vi "ReadData_6_modules.vi"(8 "error in":errorcluster, 11 "Module Config Selector":i16) -> (0 "error out":errorcluster, 1 "Number Of Pulses":u32, 2 "OversampleClk Ticks":u32, 3 "Data Array":sgl[](array[numeric]) format="%.2f")   [LabVIEW 2017, in "VDMS_VibAPI.lvlib"]
uses:
  <vilib>/addons/InsightCM/Devices/Shared/Cms/Fpga/AcquisitionFpgaTach/source/subVIs/VibAPI/VDMS_VibAPI.lvlib
  <vilib>/rvi/eio/common/nirviEmuTemplateMethod_errors.vi
  <vilib>/rvi/Memory/Memory_Emulation/nirvimemoryFastEmulation.vi
  <vilib>/rvi/Memory/Memory_Emulation/nirvimemoryEmulation.vi
  <vilib>/rvi/Emulation/niFpgaEmulationIsFPGAContextNoSignature.vi
  <vilib>/rvi/DataTransferAndStorage/Container/Common/niFpgaContainerGetUniqueNameForEmu.vi
  <vilib>/rvi/Emulation/niFpgaProcessEmulError.vi
  <vilib>/rvi/Emulation/niFpgaSctlEmulationGetInTimedLoop.vi
  <vilib>/rvi/errors/nirviReportUnexpectedCaseInternalError (U32).vi
  <vilib>/eio/EIONode/EIONode.xnode
  <vilib>/rvi/DataTransferAndStorage/Container/XNode/niFpgaContainer.xnode
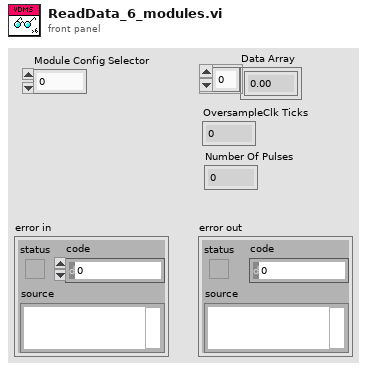
[diagram p1: front panel]
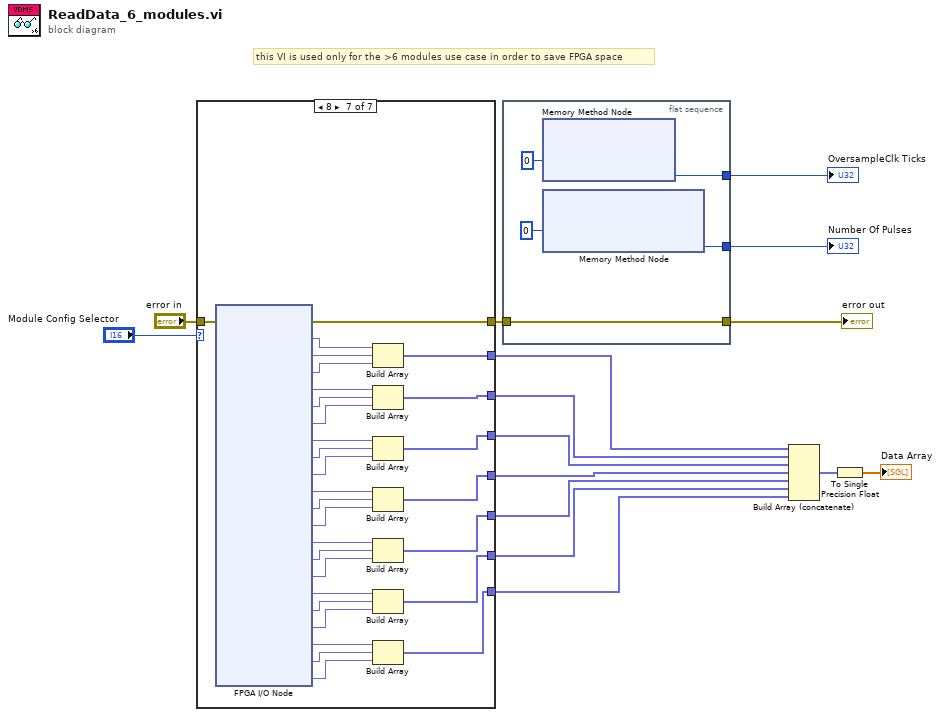
[diagram p0: block diagram]
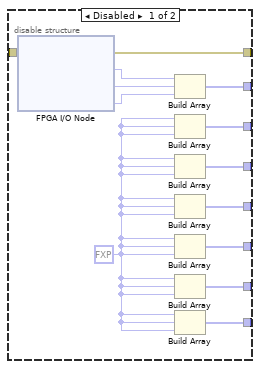
[diagram p3: hidden frame]
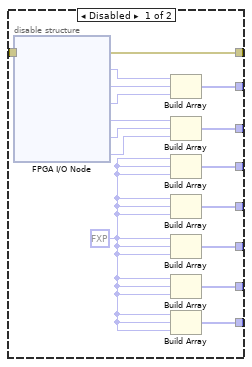
[diagram p5: hidden frame]
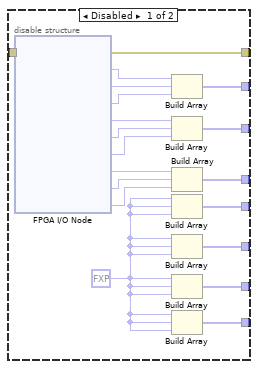
[diagram p7: hidden frame]
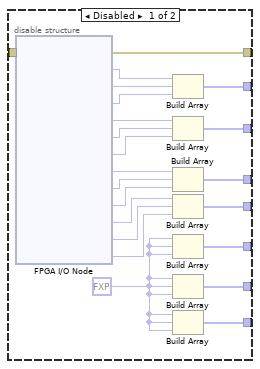
[diagram p9: hidden frame]
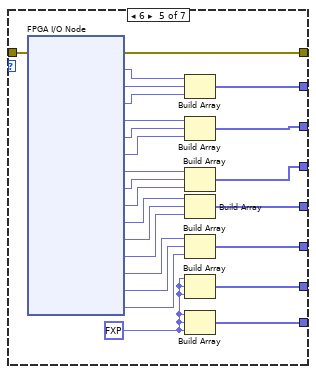
[diagram p10: hidden frame]
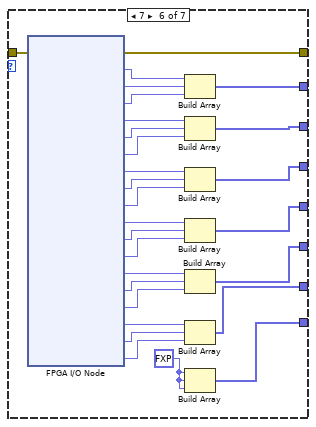
[diagram p11: hidden frame]
diagram:
  # "this VI is used only for the >6 modules use case in order to save FPGA space"
  n1 = case shown="8" "Module Config Selector" {
    tunnel: "error in" -> [w24 w47 w73 w102 w150 w178 w208]
    tunnel: [w23 w46 w72 w101 w149 w177 w207] -> w6
    tunnel: [w22 w45 w71 w100 w148 w176 w206] -> w14
    tunnel: [w21 w44 w70 w99 w147 w175 w205] -> w13
    tunnel: [w20 w43 w69 w98 w146 w174 w204] -> w12
    tunnel: [w19 w42 w68 w97 w145 w173 w203] -> w11
    tunnel: [w18 w41 w67 w96 w144 w172 w202] -> w10
    tunnel: [w17 w40 w66 w95 w143 w171 w201] -> w8
    tunnel: [w16 w39 w65 w94 w142 w170 w200] -> w7
    frame 2, Default {
      n2 = disable-structure shown="Enabled" {
        disable-tunnel: w24 -> [w37 w38]
        disable-tunnel: [w36 w38] -> w23
        disable-tunnel: [w35 _] -> w22
        disable-tunnel: [w34 _] -> w21
        disable-tunnel: [w33 _] -> w20
        disable-tunnel: [w32 _] -> w19
        disable-tunnel: [w31 _] -> w18
        disable-tunnel: [w27 _] -> w17
        disable-tunnel: [w25 _] -> w16
        frame Disabled {
          w26 = fxp<+/-,24,7> 0.0 ("Mod1/AI2")
          n3 = xnode "FPGA I/O Node"("error in"=w37) -> ("error out"=w36:errorcluster, "Mod2/AI0"=w30:fxp<+/-,24,7>, "Mod2/AI1"=w29:fxp<+/-,24,7>, "Mod2/AI2"=w28:fxp<+/-,24,7>)  [unwired: 3 in, 3 out]
          n4 = Build Array(w30, w29, w28) -> (w35:fxp<+/-,24,7>[])
          n5 = Build Array(w26, w26, w26) -> (w34:fxp<+/-,24,7>[])
          n6 = Build Array(w26, w26, w26) -> (w33:fxp<+/-,24,7>[])
          n7 = Build Array(w26, w26, w26) -> (w32:fxp<+/-,24,7>[])
          n8 = Build Array(w26, w26, w26) -> (w31:fxp<+/-,24,7>[])
          n9 = Build Array(w26, w26, w26) -> (w27:fxp<+/-,24,7>[])
          n10 = Build Array(w26, w26, w26) -> (w25:fxp<+/-,24,7>[])
        }
        frame Enabled {
        }
      }
    }
    frame 3 {
      n11 = disable-structure shown="Enabled" {
        disable-tunnel: w47 -> [w63 w64]
        disable-tunnel: [w62 w64] -> w46
        disable-tunnel: [w61 _] -> w45
        disable-tunnel: [w60 _] -> w44
        disable-tunnel: [w59 _] -> w43
        disable-tunnel: [w58 _] -> w42
        disable-tunnel: [w57 _] -> w41
        disable-tunnel: [w50 _] -> w40
        disable-tunnel: [w48 _] -> w39
        frame Disabled {
          w49 = fxp<+/-,24,7> 0.0 ("Mod1/AI2")
          n12 = xnode "FPGA I/O Node"("error in"=w63) -> ("error out"=w62:errorcluster, "Mod2/AI0"=w56:fxp<+/-,24,7>, "Mod2/AI1"=w55:fxp<+/-,24,7>, "Mod2/AI2"=w54:fxp<+/-,24,7>, "Mod3/AI0"=w53:fxp<+/-,24,7>, "Mod3/AI1"=w52:fxp<+/-,24,7>, "Mod3/AI2"=w51:fxp<+/-,24,7>)  [unwired: 6 in, 6 out]
          n13 = Build Array(w56, w55, w54) -> (w61:fxp<+/-,24,7>[])
          n14 = Build Array(w53, w52, w51) -> (w60:fxp<+/-,24,7>[])
          n15 = Build Array(w49, w49, w49) -> (w59:fxp<+/-,24,7>[])
          n16 = Build Array(w49, w49, w49) -> (w58:fxp<+/-,24,7>[])
          n17 = Build Array(w49, w49, w49) -> (w57:fxp<+/-,24,7>[])
          n18 = Build Array(w49, w49, w49) -> (w50:fxp<+/-,24,7>[])
          n19 = Build Array(w49, w49, w49) -> (w48:fxp<+/-,24,7>[])
        }
        frame Enabled {
        }
      }
    }
    frame 4 {
      n20 = disable-structure shown="Enabled" {
        disable-tunnel: w73 -> [w92 w93]
        disable-tunnel: [w91 w93] -> w72
        disable-tunnel: [w90 _] -> w71
        disable-tunnel: [w89 _] -> w70
        disable-tunnel: [w88 _] -> w69
        disable-tunnel: [w87 _] -> w68
        disable-tunnel: [w86 _] -> w67
        disable-tunnel: [w76 _] -> w66
        disable-tunnel: [w74 _] -> w65
        frame Disabled {
          w75 = fxp<+/-,24,7> 0.0 ("Mod1/AI2")
          n21 = xnode "FPGA I/O Node"("error in"=w92) -> ("error out"=w91:errorcluster, "Mod2/AI0"=w85:fxp<+/-,24,7>, "Mod2/AI1"=w84:fxp<+/-,24,7>, "Mod2/AI2"=w83:fxp<+/-,24,7>, "Mod3/AI0"=w82:fxp<+/-,24,7>, "Mod3/AI1"=w81:fxp<+/-,24,7>, "Mod3/AI2"=w80:fxp<+/-,24,7>, "Mod4/AI0"=w79:fxp<+/-,24,7>, "Mod4/AI1"=w78:fxp<+/-,24,7>, "Mod4/AI2"=w77:fxp<+/-,24,7>)  [unwired: 9 in, 9 out]
          n22 = Build Array(w85, w84, w83) -> (w90:fxp<+/-,24,7>[])
          n23 = Build Array(w82, w81, w80) -> (w89:fxp<+/-,24,7>[])
          n24 = Build Array(w79, w78, w77) -> (w88:fxp<+/-,24,7>[])
          n25 = Build Array(w75, w75, w75) -> (w87:fxp<+/-,24,7>[])
          n26 = Build Array(w75, w75, w75) -> (w86:fxp<+/-,24,7>[])
          n27 = Build Array(w75, w75, w75) -> (w76:fxp<+/-,24,7>[])
          n28 = Build Array(w75, w75, w75) -> (w74:fxp<+/-,24,7>[])
        }
        frame Enabled {
        }
      }
    }
    frame 5 {
      n29 = disable-structure shown="Enabled" {
        disable-tunnel: w102 -> [w124 w125]
        disable-tunnel: [w123 w125] -> w101
        disable-tunnel: [w122 _] -> w100
        disable-tunnel: [w121 _] -> w99
        disable-tunnel: [w120 _] -> w98
        disable-tunnel: [w119 _] -> w97
        disable-tunnel: [w118 _] -> w96
        disable-tunnel: [w117 _] -> w95
        disable-tunnel: [w116 _] -> w94
        frame Disabled {
          w103 = fxp<+/-,24,7> 0.0 ("Mod1/AI2")
          n30 = xnode "FPGA I/O Node"("error in"=w124) -> ("error out"=w123:errorcluster, "Mod2/AI0"=w115:fxp<+/-,24,7>, "Mod2/AI1"=w114:fxp<+/-,24,7>, "Mod2/AI2"=w113:fxp<+/-,24,7>, "Mod3/AI0"=w112:fxp<+/-,24,7>, "Mod3/AI1"=w111:fxp<+/-,24,7>, "Mod3/AI2"=w110:fxp<+/-,24,7>, "Mod4/AI0"=w109:fxp<+/-,24,7>, "Mod4/AI1"=w108:fxp<+/-,24,7>, "Mod4/AI2"=w107:fxp<+/-,24,7>, "Mod5/AI0"=w106:fxp<+/-,24,7>, "Mod5/AI1"=w105:fxp<+/-,24,7>, "Mod5/AI2"=w104:fxp<+/-,24,7>)  [unwired: 12 in, 12 out]
          n31 = Build Array(w115, w114, w113) -> (w122:fxp<+/-,24,7>[])
          n32 = Build Array(w112, w111, w110) -> (w121:fxp<+/-,24,7>[])
          n33 = Build Array(w109, w108, w107) -> (w120:fxp<+/-,24,7>[])
          n34 = Build Array(w106, w105, w104) -> (w119:fxp<+/-,24,7>[])
          n35 = Build Array(w103, w103, w103) -> (w118:fxp<+/-,24,7>[])
          n36 = Build Array(w103, w103, w103) -> (w117:fxp<+/-,24,7>[])
          n37 = Build Array(w103, w103, w103) -> (w116:fxp<+/-,24,7>[])
        }
        frame Enabled {
        }
      }
    }
    frame 6 {
      w126 = fxp<+/-,24,7> 0.0 ("Mod1/AI2")
      n38 = xnode "FPGA I/O Node"("error in"=w150) -> ("error out"=w149:errorcluster, "Mod2/AI0"=w141:fxp<+/-,24,7>, "Mod2/AI1"=w140:fxp<+/-,24,7>, "Mod2/AI2"=w139:fxp<+/-,24,7>, "Mod3/AI0"=w138:fxp<+/-,24,7>, "Mod3/AI1"=w137:fxp<+/-,24,7>, "Mod3/AI2"=w136:fxp<+/-,24,7>, "Mod4/AI0"=w135:fxp<+/-,24,7>, "Mod4/AI1"=w134:fxp<+/-,24,7>, "Mod4/AI2"=w133:fxp<+/-,24,7>, "Mod5/AI0"=w132:fxp<+/-,24,7>, "Mod5/AI1"=w131:fxp<+/-,24,7>, "Mod5/AI2"=w130:fxp<+/-,24,7>, "Mod6/AI0"=w129:fxp<+/-,24,7>, "Mod6/AI1"=w128:fxp<+/-,24,7>, "Mod6/AI2"=w127:fxp<+/-,24,7>)  [unwired: 15 in, 15 out]
      n39 = Build Array(w141, w140, w139) -> (w148:fxp<+/-,24,7>[])
      n40 = Build Array(w138, w137, w136) -> (w147:fxp<+/-,24,7>[])
      n41 = Build Array(w135, w134, w133) -> (w146:fxp<+/-,24,7>[])
      n42 = Build Array(w132, w131, w130) -> (w145:fxp<+/-,24,7>[])
      n43 = Build Array(w129, w128, w127) -> (w144:fxp<+/-,24,7>[])
      n44 = Build Array(w126, w126, w126) -> (w143:fxp<+/-,24,7>[])
      n45 = Build Array(w126, w126, w126) -> (w142:fxp<+/-,24,7>[])
    }
    frame 7 {
      w151 = fxp<+/-,24,7> 0.0 ("Mod1/AI2")
      n46 = xnode "FPGA I/O Node"("error in"=w178) -> ("error out"=w177:errorcluster, "Mod2/AI0"=w155:fxp<+/-,24,7>, "Mod2/AI1"=w156:fxp<+/-,24,7>, "Mod2/AI2"=w157:fxp<+/-,24,7>, "Mod3/AI0"=w158:fxp<+/-,24,7>, "Mod3/AI1"=w159:fxp<+/-,24,7>, "Mod3/AI2"=w160:fxp<+/-,24,7>, "Mod4/AI0"=w161:fxp<+/-,24,7>, "Mod4/AI1"=w162:fxp<+/-,24,7>, "Mod4/AI2"=w163:fxp<+/-,24,7>, "Mod5/AI0"=w164:fxp<+/-,24,7>, "Mod5/AI1"=w165:fxp<+/-,24,7>, "Mod5/AI2"=w166:fxp<+/-,24,7>, "Mod6/AI0"=w167:fxp<+/-,24,7>, "Mod6/AI1"=w168:fxp<+/-,24,7>, "Mod6/AI2"=w169:fxp<+/-,24,7>, "Mod7/AI0"=w154:fxp<+/-,24,7>, "Mod7/AI1"=w153:fxp<+/-,24,7>, "Mod7/AI2"=w152:fxp<+/-,24,7>)  [unwired: 18 in, 18 out]
      n47 = Build Array(w155, w156, w157) -> (w176:fxp<+/-,24,7>[])
      n48 = Build Array(w158, w159, w160) -> (w175:fxp<+/-,24,7>[])
      n49 = Build Array(w161, w162, w163) -> (w174:fxp<+/-,24,7>[])
      n50 = Build Array(w164, w165, w166) -> (w173:fxp<+/-,24,7>[])
      n51 = Build Array(w167, w168, w169) -> (w172:fxp<+/-,24,7>[])
      n52 = Build Array(w154, w153, w152) -> (w171:fxp<+/-,24,7>[])
      n53 = Build Array(w151, w151, w151) -> (w170:fxp<+/-,24,7>[])
    }
    frame 8 {
      n54 = xnode "FPGA I/O Node"("error in"=w208) -> ("error out"=w207:errorcluster, "Mod2/AI0"=w185:fxp<+/-,24,7>, "Mod2/AI1"=w186:fxp<+/-,24,7>, "Mod2/AI2"=w187:fxp<+/-,24,7>, "Mod3/AI0"=w188:fxp<+/-,24,7>, "Mod3/AI1"=w189:fxp<+/-,24,7>, "Mod3/AI2"=w190:fxp<+/-,24,7>, "Mod4/AI0"=w191:fxp<+/-,24,7>, "Mod4/AI1"=w192:fxp<+/-,24,7>, "Mod4/AI2"=w193:fxp<+/-,24,7>, "Mod5/AI0"=w194:fxp<+/-,24,7>, "Mod5/AI1"=w195:fxp<+/-,24,7>, "Mod5/AI2"=w196:fxp<+/-,24,7>, "Mod6/AI0"=w197:fxp<+/-,24,7>, "Mod6/AI1"=w198:fxp<+/-,24,7>, "Mod6/AI2"=w199:fxp<+/-,24,7>, "Mod7/AI0"=w184:fxp<+/-,24,7>, "Mod7/AI1"=w183:fxp<+/-,24,7>, "Mod7/AI2"=w182:fxp<+/-,24,7>, "Mod8/AI0"=w181:fxp<+/-,24,7>, "Mod8/AI1"=w180:fxp<+/-,24,7>, "Mod8/AI2"=w179:fxp<+/-,24,7>)  [unwired: 21 in, 21 out]
      n55 = Build Array(w185, w186, w187) -> (w206:fxp<+/-,24,7>[])
      n56 = Build Array(w188, w189, w190) -> (w205:fxp<+/-,24,7>[])
      n57 = Build Array(w191, w192, w193) -> (w204:fxp<+/-,24,7>[])
      n58 = Build Array(w194, w195, w196) -> (w203:fxp<+/-,24,7>[])
      n59 = Build Array(w197, w198, w199) -> (w202:fxp<+/-,24,7>[])
      n60 = Build Array(w184, w183, w182) -> (w201:fxp<+/-,24,7>[])
      n61 = Build Array(w181, w180, w179) -> (w200:fxp<+/-,24,7>[])
    }
  }
  n62 = flat-sequence {
    tunnel: w6 -> [w213]
    tunnel: [w213] -> w5
    tunnel: [w212] -> w2
    tunnel: [w209] -> w1
    frame #0 {
      n63 = xnode ("Memory Method Node")("Address"=u32 0) -> ("Data"=w212:u32)  [unwired: 1 in, 1 out]
      n64 = xnode ("Memory Method Node")("Address"=u32 0) -> ("Data"=w209:u32)  [unwired: 1 in, 1 out]
    }
  }
  n65 = Build Array (concatenate)(w14, w13, w12, w11, w10, w8, w7) -> (w4:fxp<+/-,24,7>[])
  n66 = To Single Precision Float(number=w4) -> (single precision float=→"Data Array":sgl[])
  "error out" <- w5
  "OversampleClk Ticks" <- w2
  "Number Of Pulses" <- w1
